vi "ECT in Run State.vi"(0 "GEA2 Reference In":refnum<k24>, 5 "Option Selection":T2={"Soil Level"=enum."Normal", "Warm Rinse"=enum."Disable", "Fabric Softener"=enum."Disable", "Extra Rinse"=enum."Disable", "Soak"=enum."Level 0", "Stain"=enum."Off", "Spin"=enum."Normal Spin", "Load Size"=enum."Precise Fill", "Dry Load Size"=enum."65535", "Load Type"=enum."Unknown", "Deep Fill"=enum."Off"}, 7 "ECT Parameters":T1={"MS to Spin Time"=0, "Target Fill Time"=238, "MS to Agitate Time"=0, "MS to Spin before Spin Time "=0, "Adaptive Drain Time"=180, "Coast to 0 Time"=60}, 11 "Error In":errorcluster) -> (4 "GEA2 Reference Out":refnum<k24>, 6 "Pass/Fail?":bool, 8 "Report Text":string, 15 "Error Out":errorcluster)   [LabVIEW 2016, in "TLMB.lvlib"]
doc: "This vi can be used to read ERD every 1 sec for user selected repeat counts."
uses:
  Projects/TLMB.lvlib
  Q:/Common/DLLs/GEA3/GeaCommunication.dll
  Common/DLLs/GEA3/GeaCommunication.dll
  Controls/Options.ctl
  Controls/ECT Parameters.ctl
  Common/LabVIEW GEA2 Toolkit/LabVIEW_GEA2_Toolkit.lvlibp/type defs/Source_Destination.ctl
  TLMB Common/type defs/Encoder Position.ctl
  Common/LabVIEW GEA2 Toolkit/LabVIEW_GEA2_Toolkit.lvlibp/type defs/ERD Write Data In.ctl
  Common/LabVIEW GEA2 Toolkit/LabVIEW_GEA2_Toolkit.lvlibp/type defs/Data Type.ctl
  TLMB Common/type defs/UI Buttons.ctl
  Common/LabVIEW GEA2 Toolkit/LabVIEW_GEA2_Toolkit.lvlibp
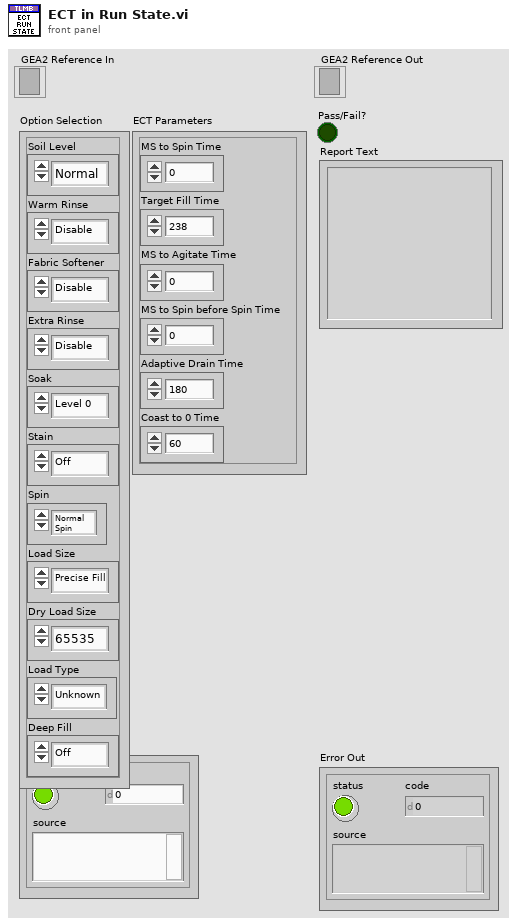
[diagram p1: front panel]
types:
  T1 = typedef "TLMB.lvlib/ECT Parameters.ctl" = cluster{"MS to Spin Time":u16, "Target Fill Time":u16, "MS to Agitate Time":u16, "MS to Spin before Spin Time ":u16, "Adaptive Drain Time":u16, "Coast to 0 Time":u16}
  T2 = typedef "TLMB.lvlib/Options.ctl" = cluster{"Soil Level":enum8{"Ex Light", "Light", "Normal", "Heavy", "Ex Heavy"}, "Warm Rinse":enum8{"Disable", "Enable"}, "Fabric Softener":enum16{"Disable", "Enable"}, "Extra Rinse":enum8{"Disable", "Enable"}, "Soak":enum8{"Level 0", "Level 1", "Level 2", "Level 3", "Level 4"}, "Stain":enum8{"Off", "Tomato", "Wine", "Blood", "Grass", "Dirt"}, "Spin":enum16{"No Spin", "Normal Spin", "More Spin", "Max Spin"}, "Load Size":enum8{"Small", "Medium", "Large", "Super", "Precise Fill", "Super Plus"}, "Dry Load Size":enum16{"128", "256", "384", "5AA", "6A4", "834", "65535"}, "Load Type":enum8{"Unknown", "Cotton", "Synthetic", "Mixed", "Wet", "Low Flow", "Small", "Medium", "Large", "Super", "Super Plus", "Max"}, "Deep Fill":enum8{"Off", "Incremental Fill", "Max Fill"}}
  T3 = typedef "LabVIEW_GEA2_Toolkit.lvlibp/Source_Destination.ctl" = cluster{"Source":u8, "Destination":u8}
  T4 = typedef "TLMB.lvlib/UI Buttons.ctl" = enum16{"Switch Off", "SW201 - My Cycle", "SW202 - Delay Wash", "SW203 - Extra Rinse", "SW204 - Signal / Volume", "SW205 - Spin", "SW206 - Deep Rinse / Fab Soft", "SW207 - Soil", "SW208 - Auto Soak", "SW209 - Temp", "SW210 - Warm Rinse", "SW211 - Deep Fill", "SW212 - Stain Remover", "SW213 - Power", "SW222 - Control Lock", "SW214 - Start / Pause", "SW301 - Start/Pause LE", "SW302 - Option Button LE", "SW201/212 - Bulk Flush"}
  T5 = typedef "LabVIEW_GEA2_Toolkit.lvlibp/ERD Write Data In.ctl" = cluster{"ERD Number":u16, "Data Type":T6, "Data":string}
  T6 = typedef "LabVIEW_GEA2_Toolkit.lvlibp/Data Type.ctl" = enum16{"string", "boolean", "uint8_t", "uint16_t", "uint32_t", "uint64_t", "int8_t", "int16_t", "int32_t", "int64_t"}
  T7 = typedef "TLMB.lvlib/Encoder Position.ctl" = enum16{"Position 0", "Position 1", "Position 2", "Position 3", "Position 4", "Position 5", "Position 6", "Position 7", "Position 8", "Position 9", "Position 10", "Position 11", "Position 12", "Position 13", "Clear / Reset"}
  T8 = typedef "TLMB.lvlib/ECT.ctl" = cluster{"MS to Agitate Time":u16, "Adaptive Drain Time":u16, "Coast to 0 Time":u16, "Agitate Time":u16, "Warm Rinse Time":u16, "FS Time":u16, "Ex Rinse Time":u16, "Soak Time":u16, "Stain Time":u16, "Motor Profile ID":u16, "Calculated ECT":u16, "Spin Time":u16}
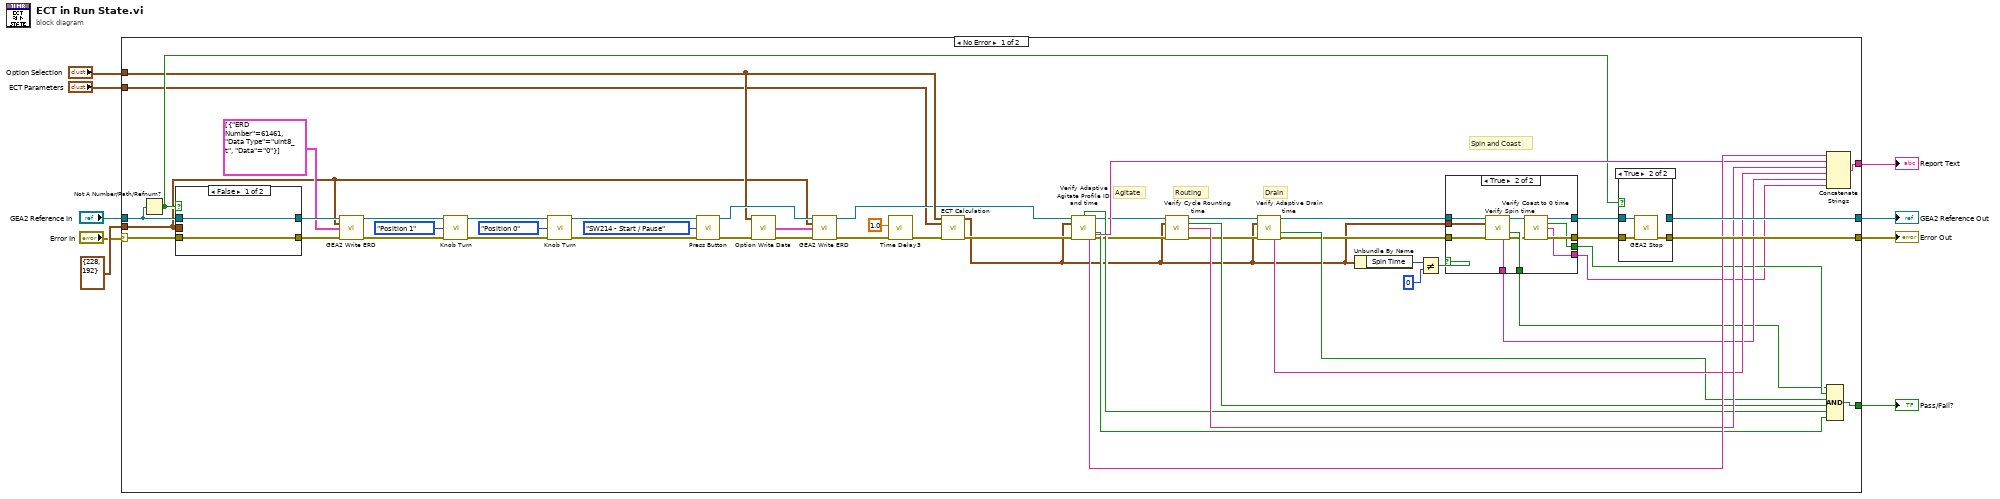
[diagram p0: block diagram]
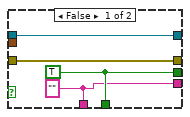
[diagram p2: hidden frame]
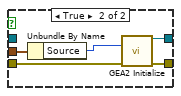
[diagram p4: hidden frame]
diagram:
  n1 = case shown="No Error" "Error In" {
    selector: "Error In" -> [w23 w92]
    tunnel: T3 {"Source"=228, "Destination"=192} ("GEA Inputs") -> [w21 _]
    tunnel: "GEA2 Reference In" -> [w64 w93]
    tunnel: [w63 w93] -> w7
    tunnel: [w62 w92] -> w6
    tunnel: "Option Selection" -> [w22 _]
    tunnel: [w56 _] -> w4
    tunnel: [w50 _] -> w3
    tunnel: "ECT Parameters" -> [w11 _]
    frame No Error {
      # "Spin and Coast"
      # "Drain"
      # "Routing"
      # "Agitate"
      n2 = Not A Number/Path/Refnum?(number/path/refnum=w64) -> (NaN/Path/Refnum?=w39:bool)
      n3 = case shown="False" w39 {
        tunnel: w23 -> [w86 w91]
        tunnel: [w86 w90] -> w44
        tunnel: [w85 w89] -> w43
        tunnel: w21 -> [_ w87]
        tunnel: w64 -> [w85 _]
        frame False {
        }
        frame True {
          n4 = Unbundle By Name(w87) -> ("Source"=w88:u8)
          n5 = call "GEA2 Initialize.vi"("Source Address"=w88, "error in"=w91) -> ("GEA2 Reference Out"=w89:refnum<k24>, "error out"=w90:errorcluster)  [unwired: 11 in, 1 out]
        }
      }
      n6 = call "GEA2 Write ERD.vi"("GEA2 Reference In"=w43, "GEA Inputs"=w21, "Write ERD List"=T5[] [{"ERD Number"=61461, "Data Type"=enum."uint8_t", "Data"="0"}], "Error In"=w44) -> ("GEA2 Reference Out"=w42:refnum<k24>, "Error Out"=w41:errorcluster)  [unwired: 9 in, 1 out]
      n7 = call "Knob Turn.vi"("GEA2 Reference In"=w42, "Knob Postiton"=Encoder_Position."Position 1" ("Button"), "Error In"=w41) -> ("GEA2 Reference Out"=w47:refnum<k24>, "Error Out"=w46:errorcluster)  [unwired: 11 in]
      n8 = call "Knob Turn.vi"("GEA2 Reference In"=w47, "Knob Postiton"=Encoder_Position."Position 0" ("Button"), "Error In"=w46) -> ("GEA2 Reference Out"=w20:refnum<k24>, "Error Out"=w19:errorcluster)  [unwired: 11 in]
      n9 = call "Press Button.vi"("GEA2 Reference In"=w20, "Button"=UI_Buttons."SW214 - Start / Pause", "Error In"=w19) -> ("GEA2 Reference Out"=w37:refnum<k24>, "Error Out"=w16:errorcluster)  [unwired: 11 in]
      n10 = call "Option Write Data.vi"("Option Selection"=w22, "Error In"=w16) -> ("appended array"=w18:T5[], "Error Out"=w17:errorcluster)  [unwired: 12 in]
      n11 = call "GEA2 Write ERD.vi"("GEA2 Reference In"=w37, "GEA Inputs"=w21, "Write ERD List"=w18, "Error In"=w17) -> ("GEA2 Reference Out"=w13:refnum<k24>, "Error Out"=w36:errorcluster)  [unwired: 9 in, 1 out]
      n12 = call "Time Delay3"("error in (no error)"=w36, "Delay Time (s)"=1.0) -> ("error out"=w35:errorcluster)  [unwired: 9 in]
      n13 = call "ECT Calculation.vi"("Option Selection"=w22, "ECT Parameters"=w11, "Error In"=w35) -> ("Expected ECT"=w10:T8, "Error Out"=w12:errorcluster)  [unwired: 11 in]
      n14 = call "Verify Adaptive Agitate Profile ID and time.vi"("GEA2 Reference In"=w13, "ECT Data In"=w10, "Error In"=w12) -> ("Motor Profile ID Pass/Fail"=w54:bool, "GEA2 Reference Out"=w34:refnum<k24>, "ECT After Agitate Pass/Fail"=w55:bool, "Agi Profile Report"=w60:string, "Report Text"=w61:string, "Error Out"=w33:errorcluster)  [unwired: 4 in, 3 out]
      n15 = call "Verify Cycle Rounting time.vi"("GEA2 Reference In"=w34, "ECT Data In"=w10, "Error In"=w33) -> ("GEA2 Reference Out"=w30:refnum<k24>, "Routing ECT pass/fail"=w53:bool, "Report Text Cycle Routing"=w59:string, "Error Out"=w32:errorcluster)  [unwired: 9 in]
      n16 = call "Verify Adaptive Drain time.vi"("GEA2 Reference In"=w30, "ECT Data In"=w10, "Error In"=w32) -> ("GEA2 Reference Out"=w29:refnum<k24>, "ECT After Drain Pass/Fail"=w49:bool, "Report Text"=w58:string, "Error Out"=w31:errorcluster)  [unwired: 6 in, 3 out]
      n17 = Unbundle By Name(w10) -> ("Spin Time"=w24:u16)
      n18 = Not Equal?(x=w24, y=u16 0) -> (x != y?=w25:bool)
      n19 = case shown="True" w25 {
        tunnel: w29 -> [w68 w79]
        tunnel: w31 -> [w67 w78]
        tunnel: [w68 w72] -> w28
        tunnel: [w67 w73] -> w27
        tunnel: [w66 w77] -> w51
        tunnel: [w65 w76] -> w57
        tunnel: [w66 w71] -> w52
        tunnel: [w65 w70] -> w14
        tunnel: w10 -> [_ w69]
        frame False {
          w66 = TRUE ("ECT After Spin Pass/Fail")
          w65 = "" ("Report Text")
        }
        frame True {
          n20 = call "Verify Spin time.vi"("GEA2 Reference In"=w79, "ECT Data In"=w69, "Error In"=w78) -> ("GEA2 Reference Out"=w74:refnum<k24>, "ECT After Spin Pass/Fail"=w77:bool, "Report Text"=w76:string, "Error Out"=w75:errorcluster)  [unwired: 6 in, 3 out]
          n21 = call "Verify Coast to 0 time.vi"("GEA2 Reference In"=w74, "Error In"=w75) -> ("GEA2 Reference Out"=w72:refnum<k24>, "Coast Pass/Fail"=w71:bool, "Report Text"=w70:string, "Error Out"=w73:errorcluster)  [unwired: 10 in]
        }
      }
      n22 = case shown="True" w39 {
        tunnel: w28 -> [w81 w84]
        tunnel: [w81 _] -> w63
        tunnel: w27 -> [w80 w83]
        tunnel: [w80 w82] -> w62
        frame False {
        }
        frame True {
          n23 = call "GEA2 Stop.vi"("GEA2 Reference In"=w84, "Error In"=w83) -> ("Error Out"=w82:errorcluster)  [unwired: 13 in]
        }
      }
      n24 = Concatenate Strings(w61, w60, w59, w58, w57, w14) -> (w56:string)
      n25 = Compound Arithmetic op=AND(w51, w52, w49, w53, w54, w55) -> (w50:bool)
    }
    frame Error {
    }
  }
  "GEA2 Reference Out" <- w7
  "Error Out" <- w6
  "Report Text" <- w4
  "Pass/Fail?" <- w3
